vi "SineWave.vi"(10 "Reset":bool, 11 "Sine Rate":i32) -> (2 "Iterator":i32, 3 "Value (0-1)":dbl)   [LabVIEW 2025, in "ArduinoSerialBling.lvlib"]
uses:
  ArduinoSerialBling.lvlib
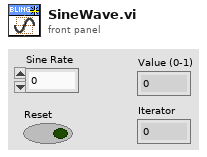
[diagram p1: front panel]
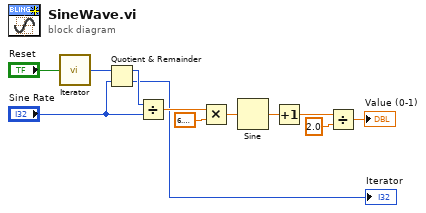
[diagram p0: block diagram]
diagram:
  n1 = call "Iterator.vi"("Reset"="Reset") -> ("i"=w3:i32)
  n2 = Quotient & Remainder(x=w3, y="Sine Rate") -> (x-y*floor(x/y)=w4:i32, floor(x/y)=→"Iterator":i32)
  n3 = Divide(x=w4, y="Sine Rate") -> (x/y=w5:dbl)
  n4 = Multiply(x=w5, y=6.283185307179586) -> (x*y=w7:dbl)
  n5 = Sine(x=w7) -> (sin(x)=w8:dbl)
  n6 = Increment(x=w8) -> (x+1=w10:dbl)
  n7 = Divide(x=w10, y=2.0) -> (x/y=→"Value (0-1)":dbl)
